vi "Remove from HashTable.vi"(8 "error in (no error)":errorcluster caption="错误输入（无错误）", 10 "Name":string, 11 "Contstant Base 输入":refnum<class "Tag Data.lvclass"> caption="DNL_LabVIEW Object in") -> (0 "error out":errorcluster caption="错误输出", 3 "Contstant Base 输出":refnum<class "Tag Data.lvclass"> caption="DNL_LabVIEW Object out")   [LabVIEW 2013, in "Tag Data.lvclass"]
uses:
  Tag Data.lvclass
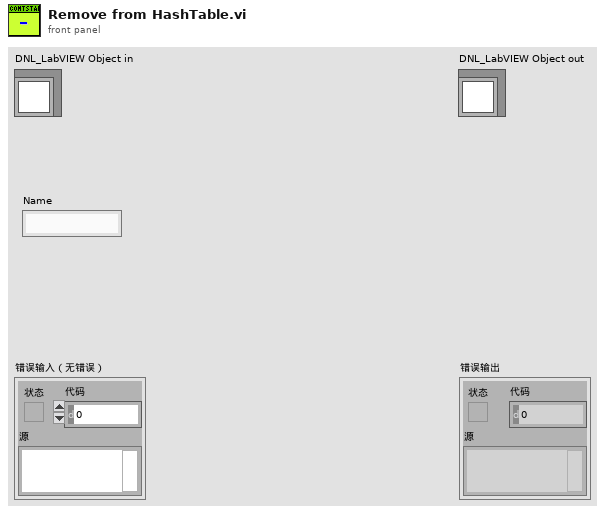
[diagram p1: front panel]
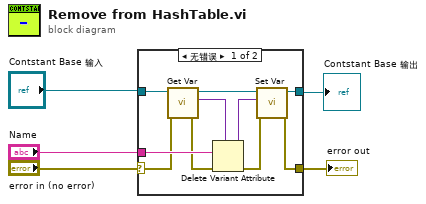
[diagram p0: block diagram]
diagram:
  n1 = case shown="无错误" "error in (no error)" {
    selector: "error in (no error)" -> [w9 w17]
    tunnel: [w6 w17] -> w4
    tunnel: [w10 w16] -> w2
    tunnel: "Contstant Base 输入" -> [w15 w16]
    tunnel: "Name" -> [w11 _]
    frame No Error {
      n2 = call-dynamic "Get Var.vi"("error in (no error)"=w9, "Contstant Base输入"=w15) -> ("error out"=w8:errorcluster, "Var"=w14:variant, "Contstant Base输出"=w12:refnum<class "Tag Data.lvclass">)  [unwired: 7 in]
      n3 = Delete Variant Attribute(4:w8, 6:w11, 7:w14) -> (0:w7:errorcluster, 3:w13:variant)  [unwired: 1 out]
      n4 = call-dynamic "Set Var.vi"("error in (no error)"=w7, "Var"=w13, "Contstant Base输入"=w12) -> ("error out"=w6:errorcluster, "Contstant Base输出"=w10:refnum<class "Tag Data.lvclass">)  [unwired: 7 in]
    }
    frame Error {
    }
  }
  "error out" <- w4
  "Contstant Base 输出" <- w2
